vi "Insert into prove.vi"(8 "error in (no error)":errorcluster, 9 "NOME NUOVA RICETTA":string, 10 "Array prove":T1(array[cluster]), 11 "Refnum in":T2) -> (0 "error out":errorcluster, 3 "Refnum out":T2)   [LabVIEW 2014]
uses:
  <vilib>/addons/database/Connection.llb/Conn ObjectReference.ctl
  <vilib>/addons/database/Connection.llb/Conn Execute.vi
  <vilib>/addons/database/Recordset.llb/Rec Destroy - Connection.vi
  <vilib>/addons/database/NI_Database_API.lvlib
panel:
  out "concatenated string":string
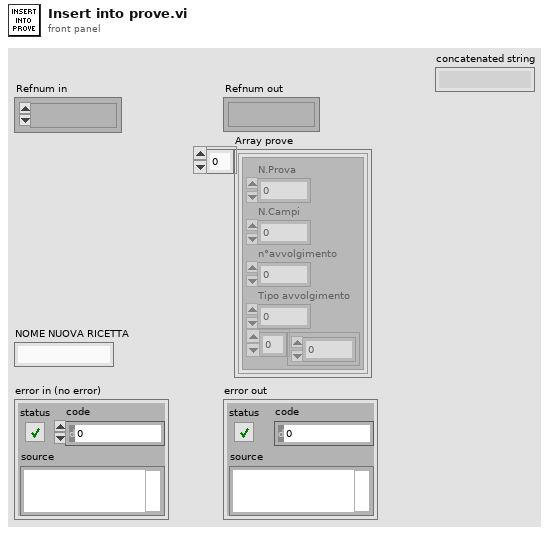
[diagram p1: front panel]
types:
  T1 = cluster{cluster{"N.Prova":i32, "N.Campi":i32, "n°avvolgimento":i16, "Tipo avvolgimento":i16, dbl[]}}[]
  T2 = typedef "NI_Database_API.lvlib/Conn ObjectReference.ctl" = refnum<k1>
  T3 = cluster{"N.Prova":i32, "N.Campi":i32, "n°avvolgimento":i16, "Tipo avvolgimento":i16, dbl[]}
  T4 = typedef "NI_Database_API.lvlib/Rec ObjectReference.ctl" = refnum<k1>
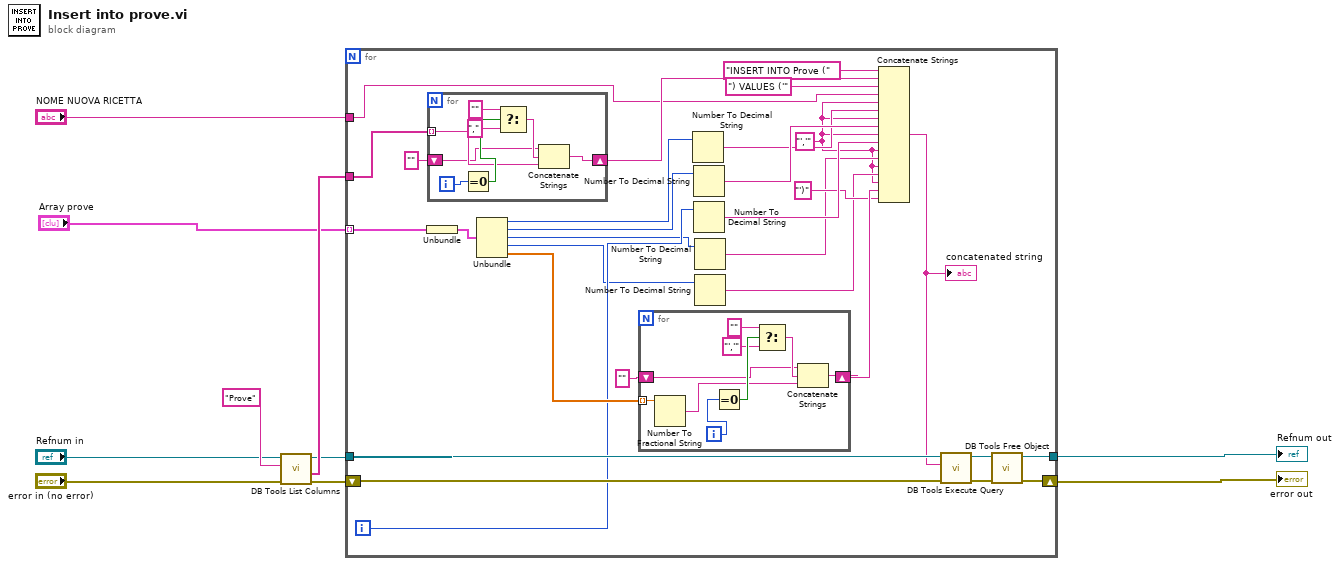
[diagram p0: block diagram]
diagram:
  n1 = call <vilib>:"DB Tools List Columns.vi"("error in (no error)"="error in (no error)", "table"="Prove", "connection reference"="Refnum in") -> ("error out"=w6:errorcluster, "columns"=w8:string[], "connection reference out"=w5:T2)  [unwired: 1 in, 1 out]
  n2 = for {
    tunnel: "NOME NUOVA RICETTA" -> [w33]
    tunnel: w8 -> [w38]
    tunnel: "Array prove" -> [w21] mode=indexing
    shift-right: [w24] -> w10
    shift-left: w6 -> [w39]
    tunnel: w5 -> [w40]
    tunnel: [w25] -> w9
    i -> [w16]
    w11 = "','" ("string")
    n3 = Unbundle(w21) -> (w20:T3)
    n4 = for {
      tunnel: w38 -> [w52] mode=indexing
      shift-right: [w51] -> w36
      shift-left: "" -> [w50]
      i -> [w57]
      n5 = Equal To 0?(x=w57) -> (x = 0?=w56:bool)
      n6 = Select(t="", s=w56, f=",") -> (s? t:f=w53:string)
      n7 = Concatenate Strings(w50, w53, w52) -> (w51:string)
    }
    n8 = Unbundle(w20) -> ("N.Prova"=w19:i32, "N.Campi"=w18:i32, "n°avvolgimento"=w15:i16, "Tipo avvolgimento"=w14:i16, w17:dbl[])
    n9 = for {
      shift-right: [w44] -> w30
      shift-left: "" -> [w43]
      tunnel: w17 -> [w41] mode=indexing
      i -> [w49]
      n10 = Number To Fractional String(number=w41) -> (F-format string=w42:string)  [unwired: 3 in]
      n11 = Equal To 0?(x=w49) -> (x = 0?=w48:bool)
      n12 = Select(t="", s=w48, f="','") -> (s? t:f=w45:string)
      n13 = Concatenate Strings(w43, w45, w42) -> (w44:string)
    }
    n14 = Number To Decimal String(number=w19) -> (decimal integer string=w22:string)  [unwired: 1 in]
    n15 = Number To Decimal String(number=w18) -> (decimal integer string=w32:string)  [unwired: 1 in]
    n16 = Number To Decimal String(number=w16) -> (decimal integer string=w31:string)  [unwired: 1 in]
    n17 = Number To Decimal String(number=w15) -> (decimal integer string=w13:string)  [unwired: 1 in]
    n18 = Number To Decimal String(number=w14) -> (decimal integer string=w12:string)  [unwired: 1 in]
    n19 = Concatenate Strings("INSERT INTO Prove (" ("SQL query"), w36, ") VALUES ('" ("string"), w33, w11, w22, w11, w32, w11, w31, w11, w13, w11, w12, w11, w30, "')" ("string")) -> (w28:string)
    "concatenated string" <- w28
    n20 = call-poly <vilib>:"DB Tools Execute Query.vi"("error in (no error)"=w39, "SQL query"=w28, "connection reference"=w40) -> ("error out"=w27:errorcluster, "recordset reference"=w26:T4)  [unwired: 5 in]
    n21 = call-poly <vilib>:"DB Tools Free Object.vi"("error in (no error)"=w27, "recordset reference"=w26) -> ("error out"=w24:errorcluster, "connection reference"=w25:T2)  [unwired: 8 in]
  }
  "error out" <- w10
  "Refnum out" <- w9
